vi "Measure.vi"(6 "error in (no error)":errorcluster, 8 "Array of Measurement to Write":dbl[](array[numeric]), 9 "Generic Data Logger in":refnum<class "Generic Data Logger.lvclass">) -> (0 "error out":errorcluster, 2 "Array of Measurement":dbl[](array[numeric]), 3 "Generic Data Logger out":refnum<class "Generic Data Logger.lvclass">)   [LabVIEW 2013, in "Generic Data Logger.lvlib" / "Generic Data Logger.lvclass"]
uses:
  Generic Data Logger.lvclass
  Generic Instrument/Generic Instrument.lvclass
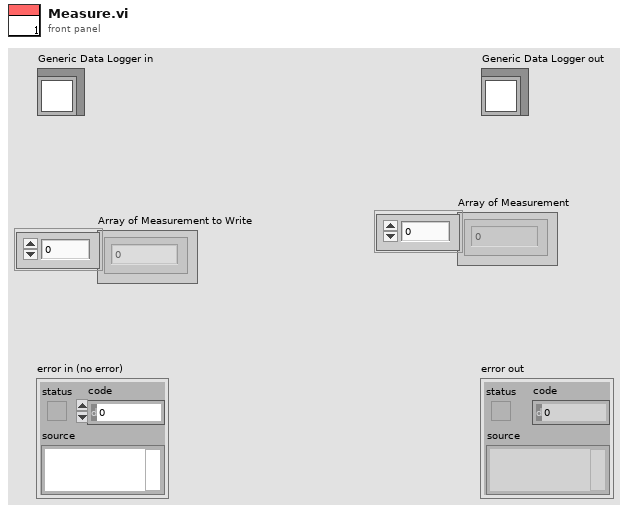
[diagram p1: front panel]
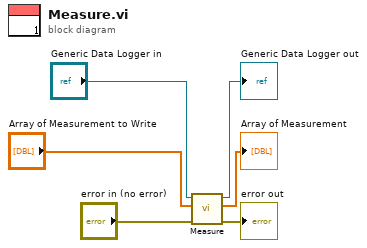
[diagram p0: block diagram]
diagram:
  n1 = call-parent "Measure.vi"("error in (no error)"="error in (no error)", "Array of Measurement to Write"="Array of Measurement to Write", "Generic Instrument in"="Generic Data Logger in") -> ("error out"=→"error out":errorcluster, "Array of Measurement"=→"Array of Measurement":dbl[], "Generic Instrument out"=→"Generic Data Logger out":refnum<class "Generic Data Logger.lvclass">)  [unwired: 4 in]
